vi "Set Measurement Options.vi"(8 "error in":errorcluster, 9 "measure Rx/Tx duration":bool, 10 "measure period":bool, 11 "data sharing framework custom device in":T1 format="%.0x") -> (0 "error out":errorcluster, 3 "data sharing framework custom device out":T1 format="%.0x")   [LabVIEW 2020, in "Data Sharing Framework Custom Device Scripting.lvlib"]
doc: "Writes the <b>measure period</b> and <b>measure Rx/Tx duration</b> options. Period and transfer duration can be used to measure and characterize performance."
uses:
  Data Sharing Framework Custom Device Scripting.lvlib
  <vilib>/NI VeriStand/Custom Device API/Custom Device Item Ref.ctl
  DSF Shared.lvlib
  <vilib>/NI VeriStand/Custom Device API/Custom Device API.lvlib
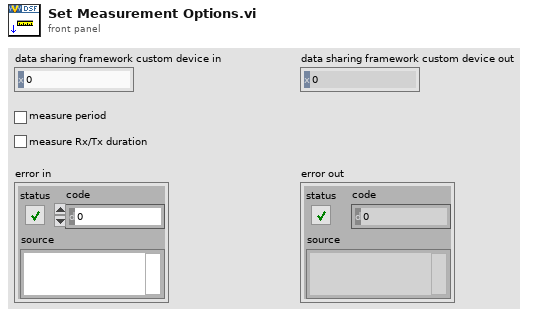
[diagram p1: front panel]
types:
  T1 = typedef "Custom Device API.lvlib/Custom Device Item Ref.ctl" = u64
  T2 = typedef "DSF Core.lvlibp/Framework.lvclass/Framework Options.ctl" = cluster{"FIFO Options":T3, "Thread Options":T4, "Plugin Options":T5, "Performance Options":T6, "Data Server Options":T7}
  T3 = typedef "DSF Core.lvlibp/Framework.lvclass/DSF FIFO Options.ctl" = cluster{"Infinite Timeouts":bool}
  T4 = typedef "DSF Core.lvlibp/Thread.lvclass/Thread Options.ctl" = cluster{"Show FP On Call":bool, "Close FP After Call":bool, "Allow Debugging":bool}
  T5 = typedef "DSF Core.lvlibp/Framework.lvclass/DSF Plugin Options.ctl" = cluster{"Default Components":bool}
  T6 = typedef "DSF Core.lvlibp/DSF Performance Options.ctl" = cluster{"Measure Period":bool, "Measure Rx/Tx Duration":bool}
  T7 = typedef "DSF Core.lvlibp/Framework.lvclass/Data Server Options.ctl" = cluster{"Enable Data Server":bool, "Period":u32}
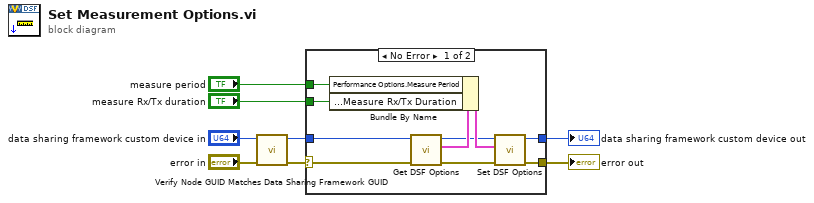
[diagram p0: block diagram]
diagram:
  n1 = call "Verify Node GUID Matches Data Sharing Framework GUID.vi"("error in"="error in", "data sharing framework custom device in"="data sharing framework custom device in") -> ("error out"=w1:errorcluster, "data sharing framework custom device out"=w2:T1)  [unwired: 8 in]
  n2 = case shown="No Error" w1 {
    selector: w1 -> [w9 w19]
    tunnel: [w18 w20] -> w8
    tunnel: [w15 w19] -> w7
    tunnel: "measure period" -> [w12 _]
    tunnel: "measure Rx/Tx duration" -> [w11 _]
    tunnel: w2 -> [w10 w20]
    frame No Error {
      n3 = call "Get DSF Options.vi"("error in (no error)"=w9, "Item Ref in"=w10) -> ("error out"=w14:errorcluster, "options"=w17:T2, "Item Ref out"=w13:T1)  [unwired: 7 in]
      n4 = Bundle By Name(cluster=w17, "Performance Options.Measure Period"=w12, "Performance Options.Measure Rx/Tx Duration"=w11) -> (w16:T2)
      n5 = call "Set DSF Options.vi"("error in (no error)"=w14, "options"=w16, "Item Ref in"=w13) -> ("error out"=w15:errorcluster, "Item Ref out"=w18:T1)  [unwired: 7 in]
    }
    frame Error {
    }
  }
  "data sharing framework custom device out" <- w8
  "error out" <- w7
